vi "read.vi"(6 "布尔":bool, 7 "写入缓冲区 2":string, 9 "写入缓冲区":string, 10 "VISA资源名称输入":refnum<visa-resource-name>, 11 "VISA引用句柄输入":refnum<visa-resource-name>) -> (2 "读取缓冲区 2":string, 3 "读取缓冲区":string)   [LabVIEW 2016]
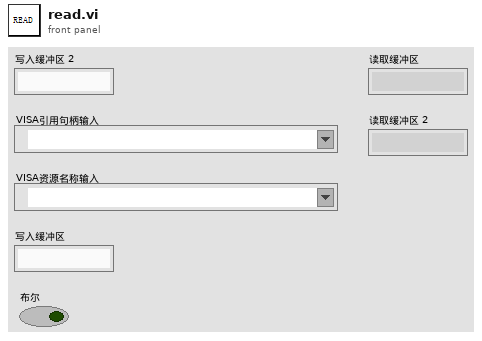
[diagram p1: front panel]
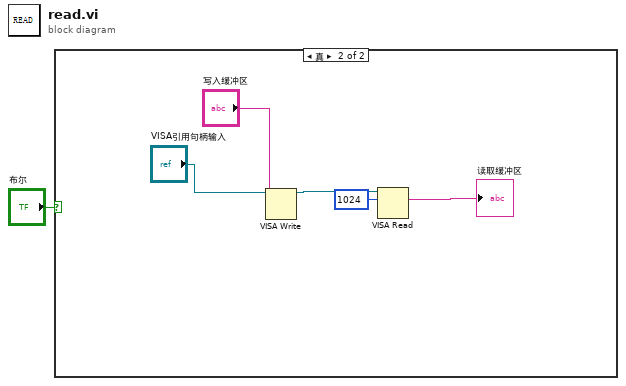
[diagram p0: block diagram]
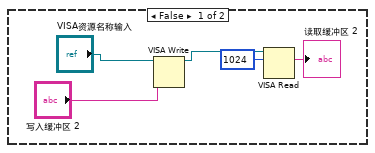
[diagram p2: hidden frame]
diagram:
  n1 = case shown="真" "布尔" {
    frame False {
      n2 = VISA Write(VISA resource name="VISA资源名称输入", write buffer="写入缓冲区 2") -> (VISA resource name out=w5:refnum<visa-resource-name>)  [unwired: 1 in, 2 out]
      n3 = VISA Read(VISA resource name=w5, byte count=u32 1024 ("字节总数")) -> (read buffer=→"读取缓冲区 2":string)  [unwired: 1 in, 3 out]
    }
    frame True {
      n4 = VISA Write(VISA resource name="VISA引用句柄输入", write buffer="写入缓冲区") -> (VISA resource name out=w10:refnum<visa-resource-name>)  [unwired: 1 in, 2 out]
      n5 = VISA Read(VISA resource name=w10, byte count=u32 1024 ("字节总数")) -> (read buffer=→"读取缓冲区":string)  [unwired: 1 in, 3 out]
    }
  }
